vi "IMU orientation.vi"(6 "Initialize ?":bool, 8 "error in (no error)":errorcluster, 9 "Yaw":sgl, 10 "Pitch":dbl, 11 "Roll":dbl) -> (0 "error out":errorcluster, 3 "3D Picture":refnum<vi>(3d-picture))   [LabVIEW 2020]
uses:
  <vilib>/picture/3D Picture Control/Object/Create Object (drawable).vi
  <vilib>/picture/3D Picture Control/Object/Add Object (no reference).vi
  <vilib>/picture/3D Picture Control/NI_3D Picture Control.lvlib
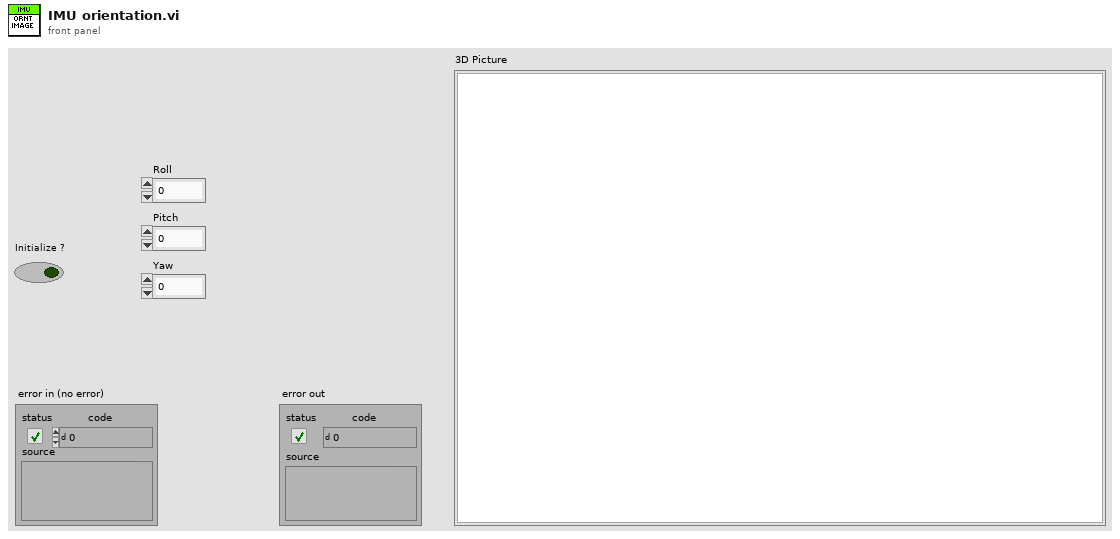
[diagram p1: front panel]
types:
  T1 = cluster{"Red":sgl, "Green":sgl, "Blue":sgl, "Alpha":sgl}
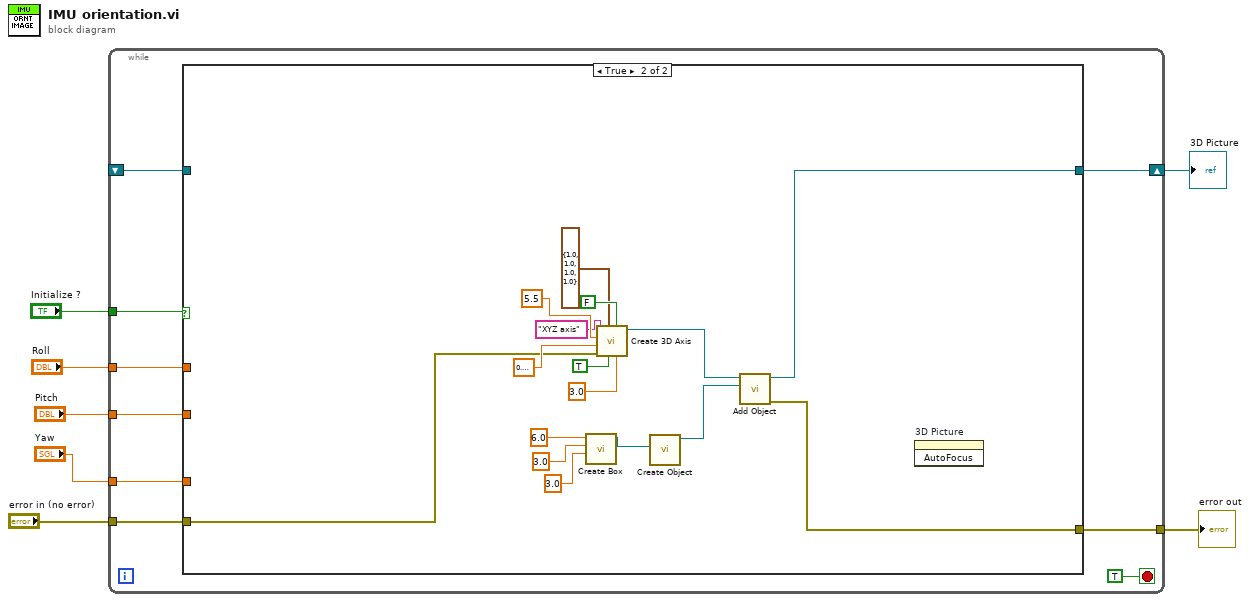
[diagram p0: block diagram]
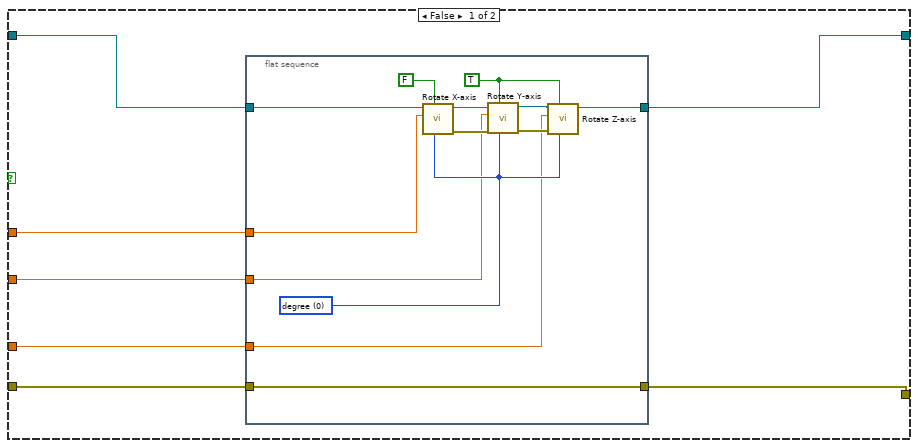
[diagram p2: hidden frame]
diagram:
  n1 = while {
    tunnel: "Initialize ?" -> [w15]
    tunnel: "error in (no error)" -> [w14]
    shift-right: [w13] -> w1
    shift-left: _ -> [w11]
    tunnel: [w12] -> w5
    tunnel: "Roll" -> [w10]
    tunnel: "Pitch" -> [w9]
    tunnel: "Yaw" -> [w8]
    stop <- TRUE stop-if-true
    n2 = case shown="True" w15 {
      tunnel: w14 -> [w21 w40]
      tunnel: [w22 w37] -> w13
      tunnel: [w20 w39] -> w12
      tunnel: w11 -> [w23 _]
      tunnel: w10 -> [w19 _]
      tunnel: w9 -> [w18 _]
      tunnel: w8 -> [w17 _]
      frame False {
        n3 = flat-sequence {
          tunnel: w23 -> [w36]
          tunnel: [w31] -> w22
          tunnel: w21 -> [w27]
          tunnel: [w27] -> w20
          tunnel: w19 -> [w26]
          tunnel: w18 -> [w25]
          tunnel: w17 -> [w24]
          frame #0 {
            w28 = TRUE ("Relative?")
            w30 = u16 0 items=["degree", "radians"] ("angle unit")
            n4 = call <vilib>:"Rotate X-axis.vi"("angle unit"=w30, "Relative?"=FALSE, "angle"=w26, "Scene Object In"=w36) -> ("error out"=w35:errorcluster, "Scene Object Out"=w33:refnum<vi>)  [unwired: 6 in]
            n5 = call <vilib>:"Rotate Y-axis.vi"("angle unit"=w30, "Relative?"=w28, "error in (no error)"=w35, "angle"=w25, "Scene Object In"=w33) -> ("error out"=w34:errorcluster, "Scene Object Out"=w32:refnum<vi>)  [unwired: 5 in]
            n6 = call <vilib>:"Rotate Z-axis.vi"("angle unit"=w30, "Relative?"=w28, "error in (no error)"=w34, "angle"=w24, "Scene Object In"=w32) -> ("Scene Object Out"=w31:refnum<vi>)  [unwired: 5 in, 1 out]
          }
        }
      }
      frame True {
        n7 = call <vilib>:"Create Box.vi"("Length Z"=sgl 3.0, "Length Y"=sgl 3.0, "Length X"=sgl 6.0) -> ("New Box Refnum"=w42:refnum<vi>)  [unwired: 7 in, 1 out]
        n8 = call <vilib>:"Create 3D Axis.vi"("Character Size"=sgl 3.0, "Half plane?"=FALSE, "Axis label?"=TRUE, "Color"=T1 {"Red"=1.0, "Green"=1.0, "Blue"=1.0, "Alpha"=1.0}, "error in (no error)"=w40, "Radius"=sgl 0.2, "Length"=sgl 5.5, "Name"="XYZ axis") -> ("New Object Refnum"=w38:refnum<vi>)  [unwired: 2 in, 1 out]
        n9 = call-poly <vilib>:"Create Object.vi"("Geometry"=w42) -> ("Scene:New Object"=w41:refnum<vi>)  [unwired: 9 in, 1 out]
        n10 = call-poly <vilib>:"Add Object.vi"("New Object In"=w41, "Scene Object In"=w38) -> ("error out"=w39:errorcluster, "Scene Object Out"=w37:refnum<vi>)  [unwired: 8 in]
        n11 = invoke on="3D Picture" class="SceneGraphDisp (strict)" method="AutoFocus"() -> ()  [unwired: 3 in, 3 out]
      }
    }
  }
  "error out" <- w5
  "3D Picture" <- w1
